vi "Teleop.vi"(10 "Match Info":T1={"Autonomous Elapsed Seconds"=0.0, "TeleOp Elapsed Seconds"=0.0, "Disabled Elapsed Seconds"=0.0, "Visited Autonomous"=FALSE, "Visited TeleOp"=FALSE, "Visited Disabled"=FALSE, "Autonomous Settings"={"Autonomous Style"=enum."Independent", "VI Refnum"=refnum}}, 11 "Call Context":T2) -> ()   [LabVIEW 2017]
doc: "This VI is called for each TeleOp packet received from the DS where the robot is not disabled. It is often used to read from the joysticks and update I/O or to update setpoints for timed control loops. It should complete and return within 20 milliseconds or it may miss DS packets."
uses:
  <vilib>/Rock Robotics/WPI/DriverStation/WPI_DriverStationDerivedRobotMode.ctl
  <vilib>/Rock Robotics/WPI/DriverStation/WPI_DriverStationMatch Info.ctl
  <vilib>/Rock Robotics/WPI/Utilities/WPI_GetSetVariantRefNum.vi
  <vilib>/Rock Robotics/Network Tables/NT Write Boolean Array.vi
  <vilib>/Rock Robotics/Network Tables/NT Write Numeric Array.vi
  <vilib>/Rock Robotics/Network Tables/NT Read Boolean.vi
  <vilib>/Rock Robotics/Network Tables/NT Read Number.vi
panel:
  out "Sample Slider 0":dbl(slide) scale=0.0..5.0
  out "Sample Boolean 1":bool
  out "Sample Boolean 0":bool
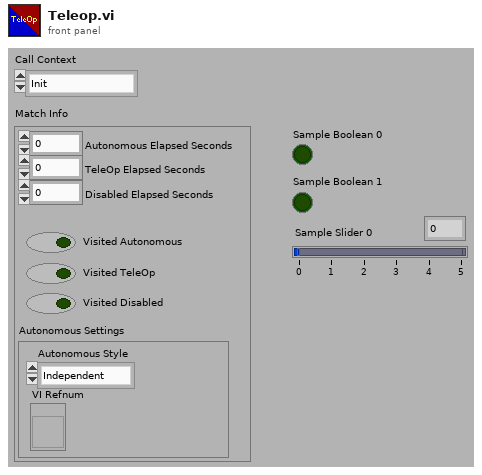
[diagram p1: front panel]
types:
  T1 = typedef "WPI_DriverStationMatch Info.ctl" = cluster{"Autonomous Elapsed Seconds":dbl, "TeleOp Elapsed Seconds":dbl, "Disabled Elapsed Seconds":dbl, "Visited Autonomous":bool, "Visited TeleOp":bool, "Visited Disabled":bool, "Autonomous Settings":cluster{"Autonomous Style":enum16{"Iterative", "Independent"}, "VI Refnum":refnum<vi>}}
  T2 = typedef "WPI_DriverStationDerivedRobotMode.ctl" = enum16{"Init", "Execute", "Stop"}
  T3 = typedef "WPI_JoystickDevRef.ctl" = cluster{"Device":T4}
  T4 = typedef "WPI_JoystickDeviceEnum.ctl" = enum16{"USB 0", "USB 1", "USB 2", "USB 3", "USB 4", "USB 5"}
  T5 = typedef "WPI_SwitchDevRef.ctl" = cluster{"DevStatus":errorcluster, "DIO Channel":T6, "CntIndex":T7, "Normally Closed":bool}
  T6 = typedef "FPGA_DIOChannel.ctl" = enum8{"DIO 0", "DIO 1", "DIO 2", "DIO 3", "DIO 4", "DIO 5", "DIO 6", "DIO 7", "DIO 8", "DIO 9", "DIO MXP 0", "DIO MXP 1", "DIO MXP 2", "DIO MXP 3", "DIO MXP 4", "DIO MXP 5", "DIO MXP 6", "DIO MXP 7", "DIO MXP 8", "DIO MXP 9", "DIO MXP 10", "DIO MXP 11", "DIO MXP 12", "DIO MXP 13", "DIO MXP 14", "DIO MXP 15", "SPI Port CS1", "SPI Port CS2", "SPI Port CS3", "SPI Port MISO", "SPI Port MOSI", "Invalid"}
  T7 = typedef "FPGA_CounterCtrSystemIndex.ctl" = enum8{"Ctr 0", "Ctr 1", "Ctr 2", "Ctr 3", "Ctr 4", "Ctr 5", "Ctr 6", "Ctr 7", "Invalid"}
  T8 = typedef "WPI_MotorControlDeviceRef.ctl" = cluster{"DeviceStatus":errorcluster, "Type":T9, "PWM":cluster{"PWM Channel":T10, "DeadBand":T11}, "CAN":cluster{"Device Number":u8, "SetOutput VI Ref":variant, "GetOutput VI Ref":variant, "Enable VI Ref":variant, "Disable VI Ref":variant, "Data":variant}, "Invert":bool, "DIO PWM":cluster{"PWM \"Enable\" Channel":T10, "DIOChannel":T6, "PWM Rate":dbl}}
  T9 = typedef "WPI_MotorControlType.ctl" = enum16{"PWM", "CAN", "DIO PWM"}
  T10 = typedef "FPGA_DIOPWMChannel.ctl" = enum8{"PWM 0", "PWM 1", "PWM 2", "PWM 3", "PWM 4", "PWM 5", "PWM 6", "PWM 7", "PWM 8", "PWM 9", "PWM MXP 0", "PWM MXP 1", "PWM MXP 2", "PWM MXP 3", "PWM MXP 4", "PWM MXP 5", "PWM MXP 6", "PWM MXP 7", "PWM MXP 8", "PWM MXP 9", "Invalid"}
  T11 = typedef "WPI_PWMDeadband.ctl" = cluster{"Name":string, "maxPositivePwm":i32, "minPositivePwm":i32, "centerPwm":i32, "maxNegativePwm":i32, "minNegativePwm":i32, "angularRange":u16}
  T12 = typedef "WPI_RobotDriveDevRef.ctl" = cluster{"DevStatus":errorcluster, "Motors[]":T8[], "Square Inputs":bool, "Max Output":dbl}
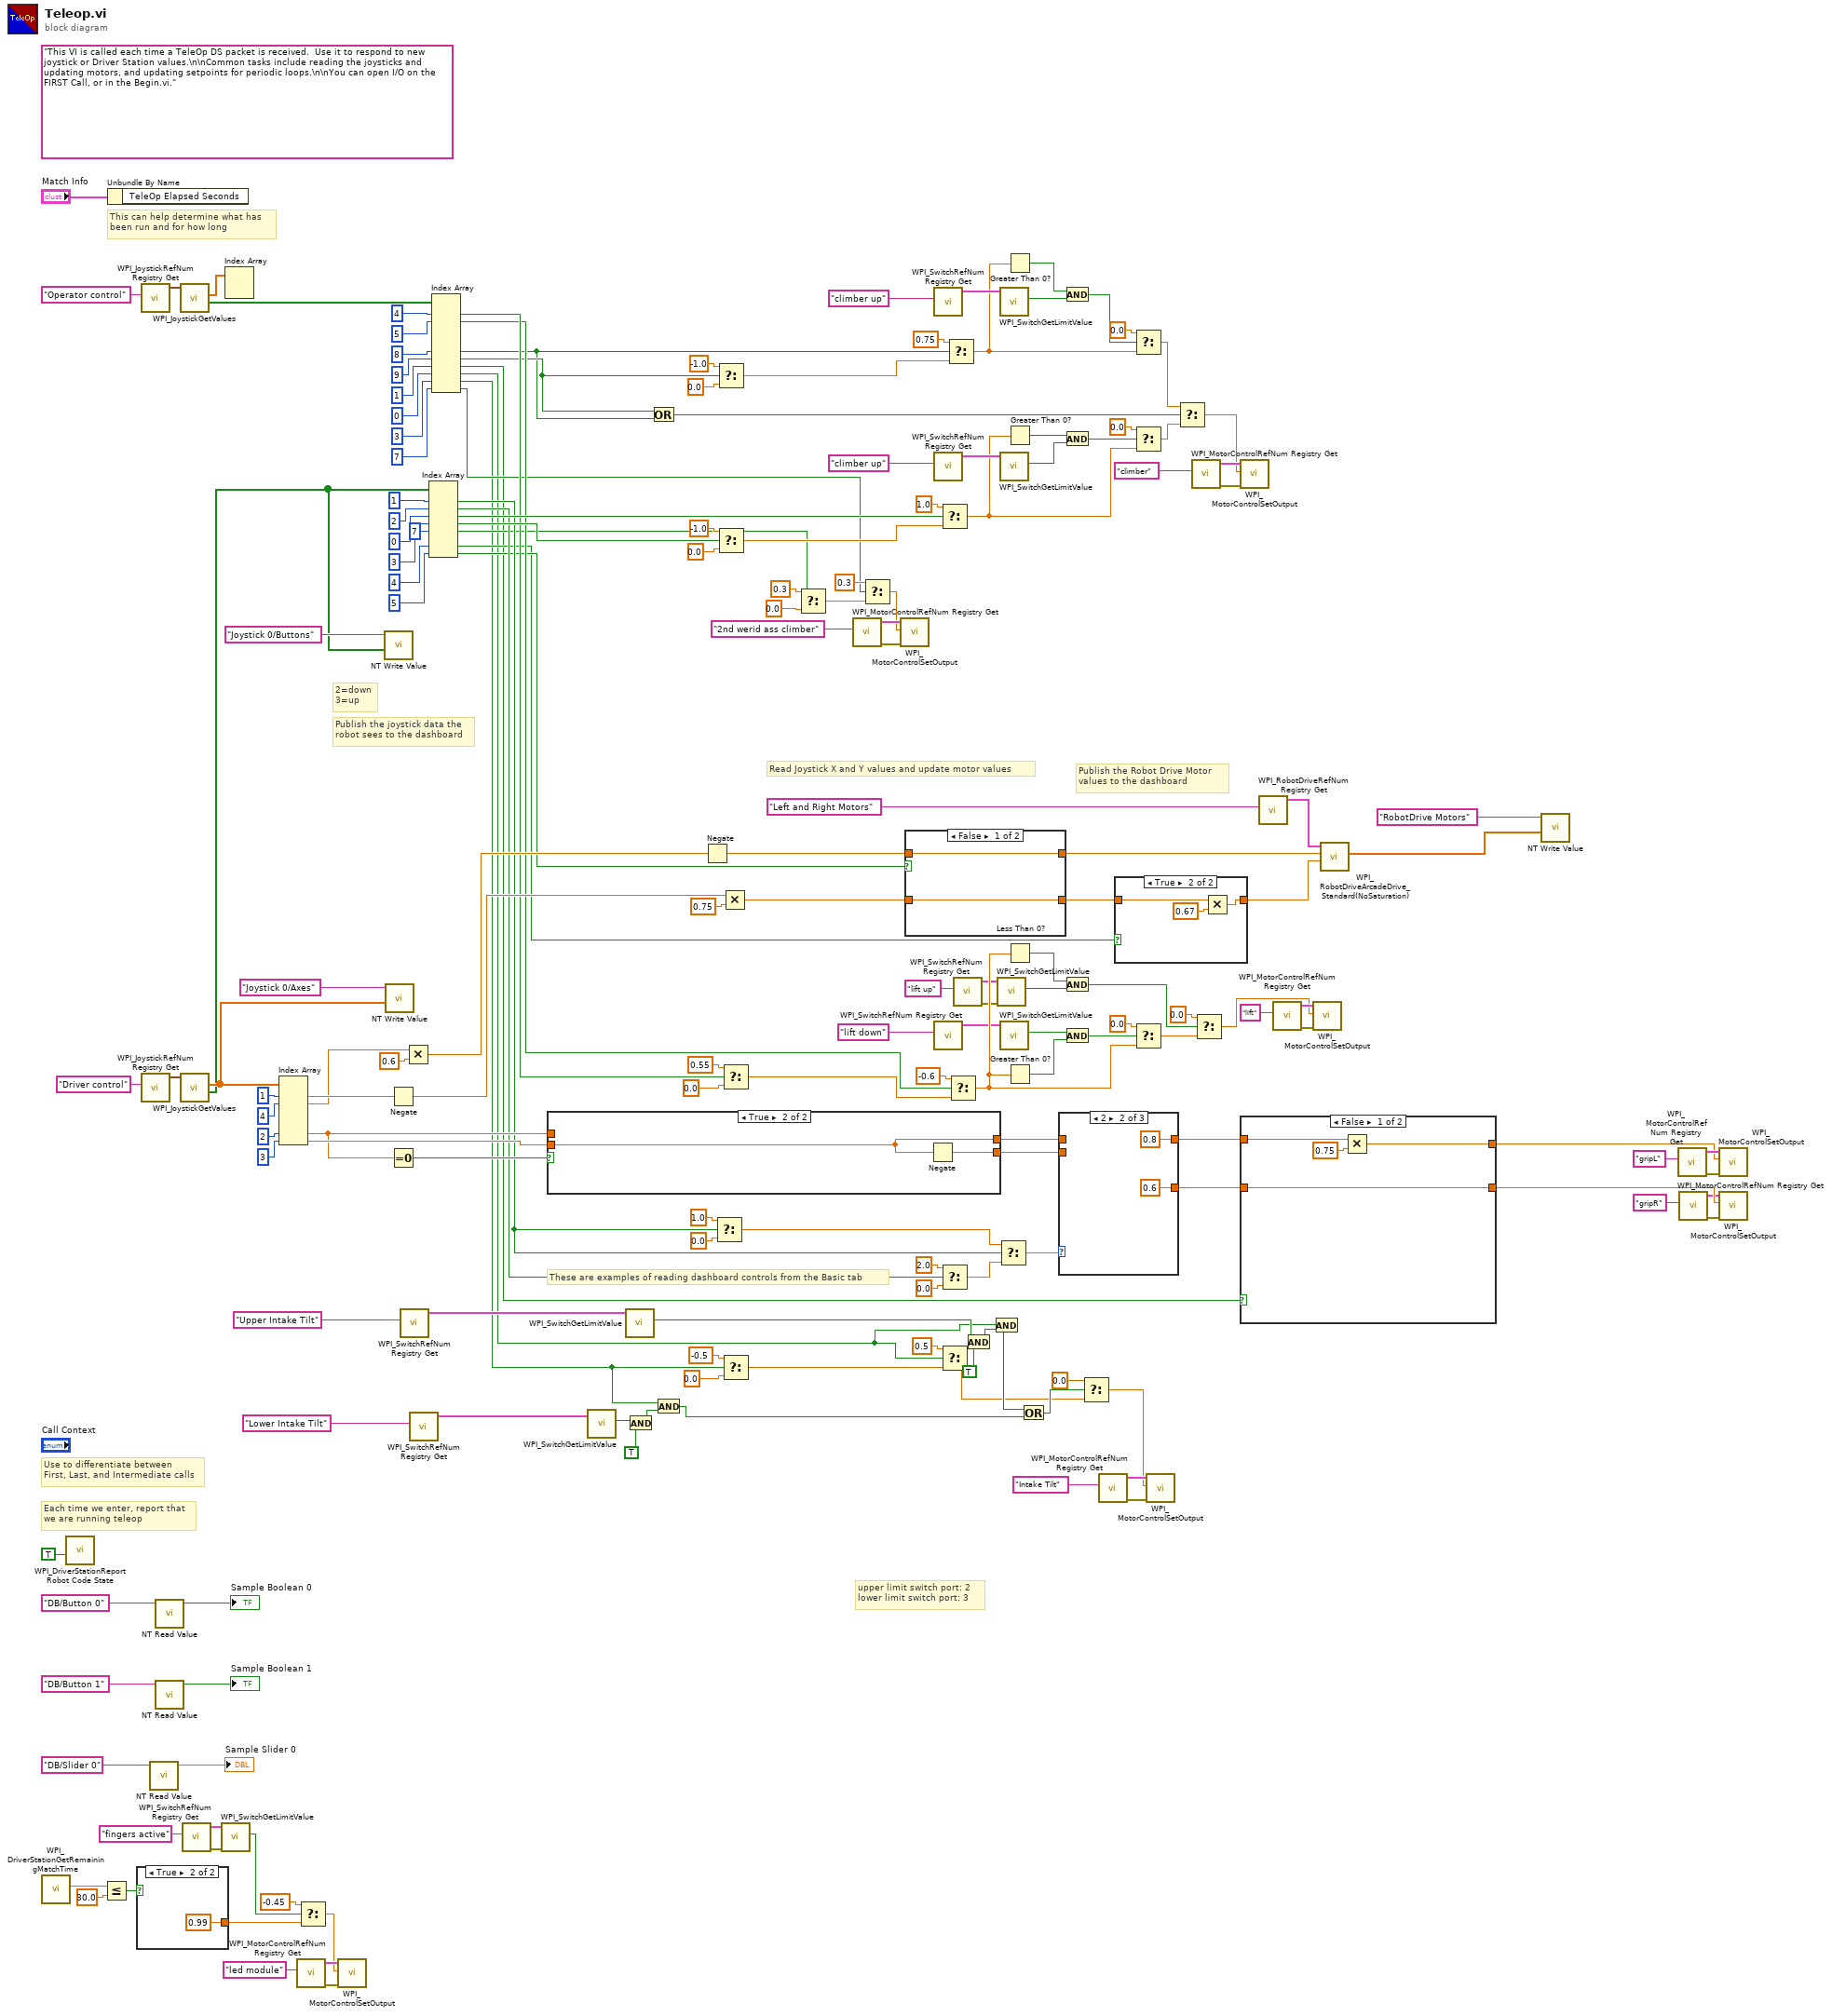
[diagram p0: block diagram]
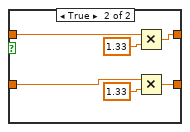
[diagram p3: hidden frame]
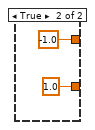
[diagram p4: hidden frame]
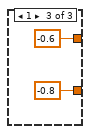
[diagram p6: hidden frame]
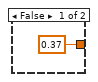
[diagram p7: hidden frame]
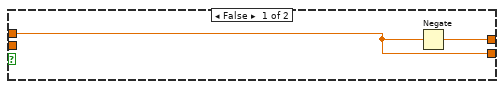
[diagram p8: hidden frame]
diagram:
  (unwired) "This VI is called each time a TeleOp DS packet is received.  Use it to respond to new joystick or Driver Station values.\n\nCommon tasks include reading the joysticks and updating motors, and updating setpoints for periodic loops.\n\nYou can open I/O on the FIRST Call, or in the Begin.vi."
  # "upper limit switch port: 2 \nlower limit switch port: 3"
  # "2=down\n3=up"
  # "These are examples of reading dashboard controls from the Basic tab"
  # "Publish the Robot Drive Motor\nvalues to the dashboard"
  # "Publish the joystick data the\nrobot sees to the dashboard"
  # "Each time we enter, report that\nwe are running teleop"
  # "Use to differentiate between\nFirst, Last, and Intermediate calls"
  # "This can help determine what has\nbeen run and for how long"
  # "Read Joystick X and Y values and update motor values"
  n1 = call <vilib>:"WPI_DriverStationGetRemainingMatchTime.vi"() -> ("Match Time(s)"=w135:sgl)  [unwired: 10 in, 1 out]
  n2 = call <vilib>:"WPI_DriverStationReport Robot Code State.vi"("TeleOp"=TRUE ("Autonomous")) -> ()  [unwired: 10 in, 1 out]
  n3 = Less Or Equal?(x=w135, y=30.0) -> (x <= y?=w134:bool)
  n4 = Unbundle By Name("Match Info") -> ()  [unwired: 1 out]
  n5 = case shown="True" w134 {
    tunnel: [0.37 0.99] -> w133
    frame False {
    }
    frame True {
    }
  }
  n6 = call <vilib>:"WPI_JoystickRefNum Registry Get.vi"("refnum name"="Operator control") -> ("JoystickDevRef"=w167:T3)  [unwired: 1 in, 9 out]
  n7 = call <vilib>:"WPI_JoystickRefNum Registry Get.vi"("refnum name"="Driver control") -> ("JoystickDevRef"=w181:T3)  [unwired: 1 in, 9 out]
  n8 = call-poly <vilib>:"NT Read Value.vi"("Name"="DB/Slider 0" ("refnum name")) -> ("Numeric"=→"Sample Slider 0":dbl)  [unwired: 9 in, 1 out]
  n9 = call-poly <vilib>:"NT Read Value.vi"("Name"="DB/Button 0" ("refnum name")) -> ("Boolean"=→"Sample Boolean 0":bool)  [unwired: 9 in, 1 out]
  n10 = call-poly <vilib>:"NT Read Value.vi"("Name"="DB/Button 1" ("refnum name")) -> ("Boolean"=→"Sample Boolean 1":bool)  [unwired: 9 in, 1 out]
  n11 = call <vilib>:"WPI_JoystickGetValues.vi"("JoystickDevRef"=w167) -> ("Buttons"=w97:bool[], "Axes"=w166:dbl[])  [unwired: 6 in, 3 out]
  n12 = call <vilib>:"WPI_JoystickGetValues.vi"("JoystickDevRef"=w181) -> ("Buttons"=w164:bool[], "Axes"=w177:dbl[])  [unwired: 6 in, 3 out]
  n13 = call <vilib>:"WPI_SwitchRefNum Registry Get.vi"("refnum name"="fingers active") -> ("error out"=w132:errorcluster, "SwitchDevRef"=w131:T5)  [unwired: 9 in]
  n14 = call <vilib>:"WPI_SwitchGetLimitValue.vi"("error in (no error)"=w132, "SwitchDevRef"=w131) -> ("Switch Pressed"=w120:bool)  [unwired: 7 in, 2 out]
  n15 = Index Array(array=w166) -> ()  [unwired: 2 in, 2 out]
  n16 = Index Array(array=w177, index #1=1 ("index"), index #2=4 ("index"), index #6=2 ("index"), index #7=3 ("index")) -> (element #1=w151:dbl, element #2=w142:dbl, element #6=w145:dbl, element #7=w146:dbl)  [unwired: 3 in, 3 out]
  n17 = call <vilib>:"WPI_MotorControlRefNum Registry Get.vi"("refnum name"="led module") -> ("error out"=w139:errorcluster, "MotorControlDevRef"=w138:T8)  [unwired: 9 in]
  n18 = Select(t=-0.45, s=w120, f=w133) -> (s? t:f=w129:dbl)
  n19 = call <vilib>:"WPI_MotorControlSetOutput.vi"("error in (no error)"=w139, "Output"=w129, "MotorControlDevRef"=w138) -> ()  [unwired: 6 in, 3 out]
  n20 = call-poly <vilib>:"NT Write Value.vi"("Boolean Array"=w164, "Name"="Joystick 0/Buttons") -> ()  [unwired: 9 in, 1 out]
  n21 = call-poly <vilib>:"NT Write Value.vi"("Numeric Array"=w177, "Name"="Joystick 0/Axes") -> ()  [unwired: 9 in, 1 out]
  n22 = Negate(x=w151) -> (-x=w144:dbl)
  n23 = Equal To 0?(x=w145) -> (x = 0?=w147:bool)
  n24 = call <vilib>:"WPI_SwitchRefNum Registry Get.vi"("refnum name"="Upper Intake Tilt") -> ("SwitchDevRef"=w37:T5)  [unwired: 9 in, 1 out]
  n25 = Multiply(x=w142, y=0.6) -> (x*y=w140:dbl)
  n26 = call <vilib>:"WPI_SwitchRefNum Registry Get.vi"("refnum name"="Lower Intake Tilt") -> ("SwitchDevRef"=w15:T5)  [unwired: 9 in, 1 out]
  n27 = Index Array(array=w164, index #1=1 ("index"), index #2=2 ("index"), index #3=0 ("index"), index #4=3 ("index"), index #5=7 ("index"), index #7=4 ("index"), index #8=5 ("index")) -> (element #1=w58:bool, element #2=w61:bool, element #3=w152:bool, element #4=w159:bool, element #5=w18:bool, element #7=w43:bool, element #8=w47:bool)  [unwired: 1 in, 1 out]
  n28 = Index Array(array=w97, index #1=4 ("index"), index #2=5 ("index"), index #6=8 ("index"), index #7=9 ("index"), index #8=1 ("index"), index #9=0 ("index"), index #10=3 ("index"), index #11=7 ("index")) -> (element #1=w94:bool, element #2=w93:bool, element #6=w74:bool, element #7=w75:bool, element #8=w17:bool, element #9=w6:bool, element #10=w14:bool, element #11=w22:bool)  [unwired: 3 in, 3 out]
  n29 = case shown="True" w147 {
    tunnel: [w189 w191] -> w56
    tunnel: w146 -> [_ w191]
    tunnel: w145 -> [w188 _]
    tunnel: [w188 w190] -> w55
    frame False {
      n30 = Negate(x=w188) -> (-x=w189:dbl)
    }
    frame True {
      n31 = Negate(x=w191) -> (-x=w190:dbl)
    }
  }
  n32 = call <vilib>:"WPI_SwitchGetLimitValue.vi"("SwitchDevRef"=w15) -> ("Switch Pressed"=w13:bool)  [unwired: 8 in, 2 out]
  n33 = call <vilib>:"WPI_SwitchGetLimitValue.vi"("SwitchDevRef"=w37) -> ("Switch Pressed"=w7:bool)  [unwired: 8 in, 2 out]
  n34 = And(x=w13, y=TRUE) -> (x .and. y?=w11:bool)
  n35 = Or(x=w75, y=w74) -> (x .or. y?=w73:bool)
  n36 = And(x=w14, y=w11) -> (x .and. y?=w10:bool)
  n37 = Negate(x=w140) -> (-x=w42:dbl)
  n38 = Select(t=1.0, s=w58, f=0.0) -> (s? t:f=w63:dbl)
  n39 = Select(t=-1.0, s=w75, f=0.0) -> (s? t:f=w87:dbl)
  n40 = Select(t=-1.0, s=w159, f=0.0) -> (s? t:f=w156:dbl)
  n41 = Multiply(x=w144, y=0.75) -> (x*y=w46:dbl)
  n42 = Select(t=0.55, s=w94, f=0.0) -> (s? t:f=w114:dbl)
  n43 = Select(t=-0.5, s=w14, f=0.0) -> (s? t:f=w34:dbl)
  n44 = Select(t=0.3, s=w18, f=0.0) -> (s? t:f=w21:dbl)
  n45 = call <vilib>:"WPI_MotorControlRefNum Registry Get.vi"("refnum name"="2nd werid ass climber") -> ("error out"=w28:errorcluster, "MotorControlDevRef"=w27:T8)  [unwired: 9 in]
  n46 = Select(t=0.3, s=w22, f=w21) -> (s? t:f=w25:dbl)
  n47 = call <vilib>:"WPI_MotorControlSetOutput.vi"("error in (no error)"=w28, "Output"=w25, "MotorControlDevRef"=w27) -> ()  [unwired: 6 in, 3 out]
  n48 = case shown="False" w47 {
    tunnel: w46 -> [w193 w199]
    tunnel: [w193 w197] -> w45
    tunnel: w42 -> [w192 w195]
    tunnel: [w192 w194] -> w41
    frame False {
    }
    frame True {
      n49 = Multiply(x=w195, y=1.33) -> (x*y=w194:dbl)
      n50 = Multiply(x=w199, y=1.33) -> (x*y=w197:dbl)
    }
  }
  n51 = call <vilib>:"WPI_SwitchRefNum Registry Get.vi"("refnum name"="climber up") -> ("SwitchDevRef"=w85:T5)  [unwired: 9 in, 1 out]
  n52 = call <vilib>:"WPI_SwitchRefNum Registry Get.vi"("refnum name"="climber up") -> ("SwitchDevRef"=w127:T5)  [unwired: 9 in, 1 out]
  n53 = call <vilib>:"WPI_SwitchRefNum Registry Get.vi"("refnum name"="lift down") -> ("SwitchDevRef"=w101:T5)  [unwired: 9 in, 1 out]
  n54 = Select(t=1.0, s=w152, f=w156) -> (s? t:f=w121:dbl)
  n55 = Select(t=2.0, s=w61, f=0.0) -> (s? t:f=w62:dbl)
  n56 = Select(t=0.5, s=w6, f=w34) -> (s? t:f=w2:dbl)
  n57 = Select(t=0.75, s=w74, f=w87) -> (s? t:f=w79:dbl)
  n58 = Select(t=-0.6, s=w93, f=w114) -> (s? t:f=w105:dbl)
  n59 = call <vilib>:"WPI_SwitchRefNum Registry Get.vi"("refnum name"="lift up") -> ("error out"=w103:errorcluster, "SwitchDevRef"=w102:T5)  [unwired: 9 in]
  n60 = And(x=w7, y=TRUE) -> (x .and. y?=w8:bool)
  n61 = And(x=w6, y=w8) -> (x .and. y?=w5:bool)
  n62 = call <vilib>:"WPI_SwitchGetLimitValue.vi"("error in (no error)"=w103, "SwitchDevRef"=w102) -> ("Switch Pressed"=w99:bool)  [unwired: 7 in, 2 out]
  n63 = Select(t=w63, s=w58, f=w62) -> (s? t:f=w57:dbl)
  n64 = call <vilib>:"WPI_SwitchGetLimitValue.vi"("SwitchDevRef"=w85) -> ("Switch Pressed"=w83:bool)  [unwired: 8 in, 2 out]
  n65 = call <vilib>:"WPI_SwitchGetLimitValue.vi"("SwitchDevRef"=w127) -> ("Switch Pressed"=w125:bool)  [unwired: 8 in, 2 out]
  n66 = call <vilib>:"WPI_SwitchGetLimitValue.vi"("SwitchDevRef"=w101) -> ("Switch Pressed"=w98:bool)  [unwired: 8 in, 2 out]
  n67 = Greater Than 0?(x=w79) -> (x > 0?=w82:bool)
  n68 = Greater Than 0?(x=w121) -> (x > 0?=w124:bool)
  n69 = Less Than 0?(x=w105) -> (x < 0?=w109:bool)
  n70 = Greater Than 0?(x=w105) -> (x > 0?=w110:bool)
  n71 = Or(x=w5, y=w10) -> (x .or. y?=w4:bool)
  n72 = case shown="2" w57 {
    tunnel: [w201 0.8 ("upper limit") -0.6 ("upper limit")] -> w52
    tunnel: w56 -> [w201 _ _]
    tunnel: [w200 0.6 ("upper limit") -0.8 ("upper limit")] -> w50
    tunnel: w55 -> [w200 _ _]
    frame 0, Default {
    }
    frame 2 {
    }
    frame 1 {
    }
  }
  n73 = And(x=w82, y=w83) -> (x .and. y?=w80:bool)
  n74 = And(x=w124, y=w125) -> (x .and. y?=w122:bool)
  n75 = And(x=w109, y=w99) -> (x .and. y?=w111:bool)
  n76 = And(x=w98, y=w110) -> (x .and. y?=w112:bool)
  n77 = Select(t=0.0, s=w4, f=w2) -> (s? t:f=w1:dbl)
  n78 = call <vilib>:"WPI_MotorControlRefNum Registry Get.vi"("refnum name"="Intake Tilt") -> ("error out"=w39:errorcluster, "MotorControlDevRef"=w40:T8)  [unwired: 9 in]
  n79 = case shown="True" w43 {
    tunnel: w45 -> [w206 w209]
    tunnel: [w206 w207] -> w44
    frame False {
    }
    frame True {
      n80 = Multiply(x=w209, y=0.67) -> (x*y=w207:dbl)
    }
  }
  n81 = Select(t=0.0, s=w80, f=w79) -> (s? t:f=w72:dbl)
  n82 = Select(t=0.0, s=w122, f=w121) -> (s? t:f=w71:dbl)
  n83 = Select(t=0.0, s=w112, f=w105) -> (s? t:f=w106:dbl)
  n84 = call <vilib>:"WPI_MotorControlSetOutput.vi"("error in (no error)"=w39, "Output"=w1, "MotorControlDevRef"=w40) -> ()  [unwired: 6 in, 3 out]
  n85 = Select(t=w72, s=w73, f=w71) -> (s? t:f=w70:dbl)
  n86 = call <vilib>:"WPI_MotorControlRefNum Registry Get.vi"("refnum name"="climber") -> ("error out"=w90:errorcluster, "MotorControlDevRef"=w91:T8)  [unwired: 9 in]
  n87 = Select(t=0.0, s=w111, f=w106) -> (s? t:f=w104:dbl)
  n88 = call <vilib>:"WPI_MotorControlSetOutput.vi"("error in (no error)"=w90, "Output"=w70, "MotorControlDevRef"=w91) -> ()  [unwired: 6 in, 3 out]
  n89 = case shown="False" w17 {
    tunnel: [w210 -1.0 ("upper limit")] -> w53
    tunnel: w52 -> [w212 _]
    tunnel: [w213 1.0 ("upper limit")] -> w51
    tunnel: w50 -> [w213 _]
    frame False {
      n90 = Multiply(x=w212, y=0.75) -> (x*y=w210:dbl)
    }
    frame True {
    }
  }
  n91 = call <vilib>:"WPI_RobotDriveRefNum Registry Get.vi"("refnum name"="Left and Right Motors") -> ("RobotDriveDevRef"=w183:T12)  [unwired: 1 in, 9 out]
  n92 = call <vilib>:"WPI_MotorControlRefNum Registry Get.vi"("refnum name"="lift") -> ("error out"=w117:errorcluster, "MotorControlDevRef"=w118:T8)  [unwired: 9 in]
  n93 = call <vilib>:"WPI_MotorControlSetOutput.vi"("error in (no error)"=w117, "Output"=w104, "MotorControlDevRef"=w118) -> ()  [unwired: 6 in, 3 out]
  n94 = call <vilib>:"WPI_RobotDriveArcadeDrive_Standard(NoSaturation).vi"("Y axis value"=w44, "X axis value"=w41, "RobotDriveDevRef"=w183) -> ("Motor Values"=w170:dbl[])  [unwired: 1 in, 7 out]
  n95 = call-poly <vilib>:"NT Write Value.vi"("Numeric Array"=w170, "Name"="RobotDrive Motors") -> ()  [unwired: 9 in, 1 out]
  n96 = call <vilib>:"WPI_MotorControlRefNum Registry Get.vi"("refnum name"="gripL") -> ("error out"=w148:errorcluster, "MotorControlDevRef"=w149:T8)  [unwired: 9 in]
  n97 = call <vilib>:"WPI_MotorControlRefNum Registry Get.vi"("refnum name"="gripR") -> ("error out"=w69:errorcluster, "MotorControlDevRef"=w49:T8)  [unwired: 9 in]
  n98 = call <vilib>:"WPI_MotorControlSetOutput.vi"("error in (no error)"=w148, "Output"=w53, "MotorControlDevRef"=w149) -> ()  [unwired: 6 in, 3 out]
  n99 = call <vilib>:"WPI_MotorControlSetOutput.vi"("error in (no error)"=w69, "Output"=w51, "MotorControlDevRef"=w49) -> ()  [unwired: 6 in, 3 out]
